vi "Append Properties to Edit Context Menu.vi"(9 "State":T1, 11 "Menu in":refnum<k9>) -> ()   [LabVIEW 2020, in "Level (G3).xctl"]
uses:
  Level (G3).xctl
  State.ctl
  Utility VIs/Controls/KRing/KRing.xctl
  Utility VIs/Controls/KNumeric (DBL)/KNumeric (DBL).xctl
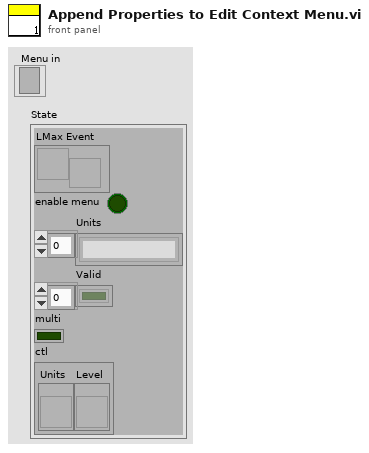
[diagram p1: front panel]
types:
  T1 = typedef "Level (G3).xctl/State.ctl" = cluster{"LMax Event":refnum<user-event>, "enable menu":bool, "Units":string[], "Valid":bool[], "multi":bool, "ctl":cluster{"Units":refnum<vi>, "Level":refnum<vi>}}
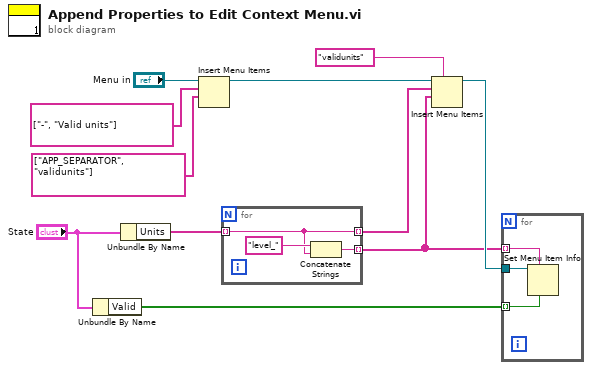
[diagram p0: block diagram]
diagram:
  n1 = Unbundle By Name("State") -> ("Valid"=w1:bool[])
  n2 = Unbundle By Name("State") -> ("Units"=w5:string[])
  n3 = Insert Menu Items(7:string[] ["APP_SEPARATOR", "validunits"] ("item names"), 8:string[] ["-", "Valid units"] ("item names"), 9:"Menu in") -> (3:w10:refnum<k9>)  [unwired: 3 in, 2 out]
  n4 = for {
    tunnel: w5 -> [w13] mode=indexing
    tunnel: [w13] -> w4 mode=indexing
    tunnel: [w12] -> w3 mode=indexing
    n5 = Concatenate Strings("level_" ("string"), w13) -> (w12:string)
  }
  n6 = Insert Menu Items(5:"validunits", 7:w3, 8:w4, 9:w10) -> (3:w6:refnum<k9>)  [unwired: 2 in, 2 out]
  n7 = for {
    tunnel: w6 -> [w17]
    tunnel: w3 -> [w16] mode=indexing
    tunnel: w1 -> [w15] mode=indexing
    n8 = Set Menu Item Info(6:w15, 7:w16, 11:w17) -> ()  [unwired: 4 in, 2 out]
  }
